vi "Insert CVT Data Core.vi"(4 "Data":variant, 5 "Nested Group":string, 6 "Nested?":bool, 7 "error in":errorcluster, 8 "tag":string, 9 "Group":string, 10 "CVT In":variant) -> (0 "error out":errorcluster, 3 "CVT Out":variant)   [LabVIEW 2014, in "Controller.lvlib" / "Controller.lvclass"]
uses:
  Controller.lvclass
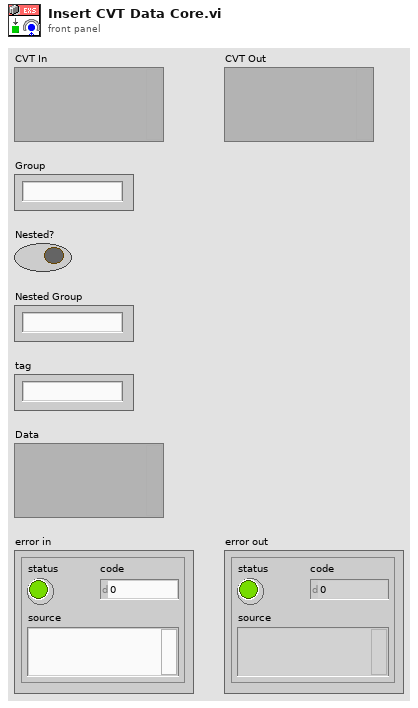
[diagram p1: front panel]
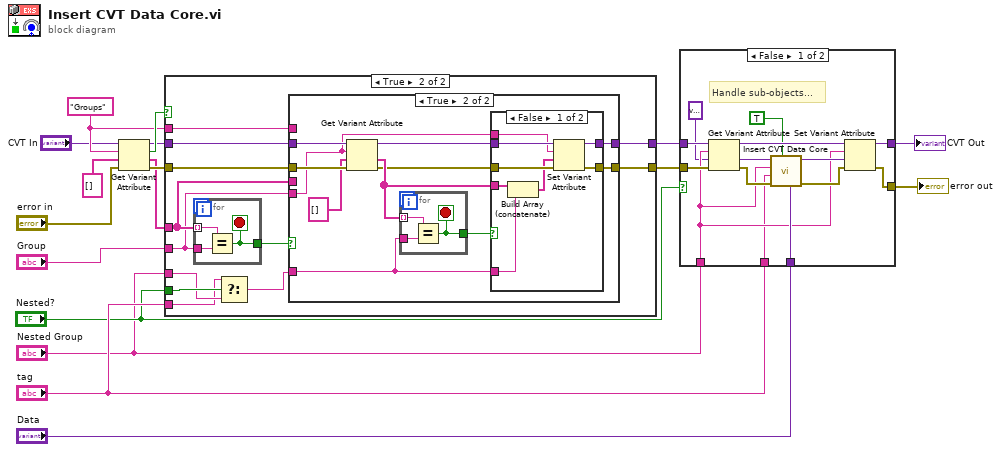
[diagram p0: block diagram]
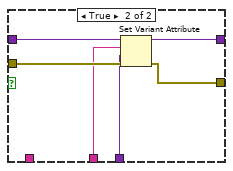
[diagram p2: hidden frame]
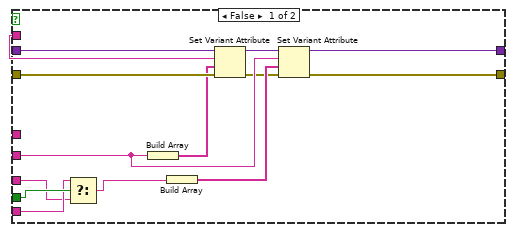
[diagram p3: hidden frame]
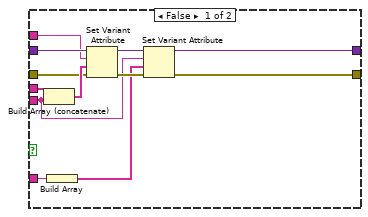
[diagram p4: hidden frame]
diagram:
  w7 = "Groups" ("name")
  n1 = Get Variant Attribute(Variant="CVT In", name=w7, default value (empty Variant)=string[] [], error in="error in") -> (duplicate Variant=w4:variant, found=w15:bool, value=w5:string[], error out=w8:errorcluster)
  n2 = case shown="True" w15 {
    tunnel: w4 -> [w31 w42]
    tunnel: w5 -> [_ w41]
    tunnel: "Group" -> [w25 w40]
    tunnel: w7 -> [w29 w39]
    tunnel: w8 -> [w30 w38]
    tunnel: [w26 w37] -> w9
    tunnel: [w23 w36] -> w10
    tunnel: "tag" -> [w20 w33]
    tunnel: "Nested?" -> [w21 w35]
    tunnel: "Nested Group" -> [w19 w34]
    frame False {
      n3 = Select(t=w20, s=w21, f=w19) -> (s? t:f=w18:string)
      n4 = Build Array(w25) -> (w28:string[])
      n5 = Build Array(w18) -> (w24:string[])
      n6 = Set Variant Attribute(Variant=w31, name=w29, value=w28, error in=w30) -> (Variant out=w27:variant, error out=w22:errorcluster)  [unwired: 1 out]
      n7 = Set Variant Attribute(Variant=w27, name=w25, value=w24, error in=w22) -> (Variant out=w26:variant, error out=w23:errorcluster)  [unwired: 1 out]
    }
    frame True {
      n8 = for {
        tunnel: w41 -> [w81] mode=indexing
        tunnel: w40 -> [w82]
        tunnel: [w80] -> w43
        stop <- w80 stop-if-true
        n9 = Equal?(x=w81, y=w82) -> (x = y?=w80:bool)
      }
      n10 = Select(t=w33, s=w35, f=w34) -> (s? t:f=w32:string)
      n11 = case shown="True" w43 {
        tunnel: w42 -> [w55 w66]
        tunnel: w41 -> [w54 _]
        tunnel: w40 -> [w48 w56]
        tunnel: w39 -> [w52 _]
        tunnel: [w45 w57] -> w37
        tunnel: [w44 w58] -> w36
        tunnel: w38 -> [w51 w65]
        tunnel: w32 -> [w47 w60]
        frame False {
          n12 = Build Array (concatenate)(w54, w48) -> (w53:string[])
          n13 = Build Array(w47) -> (w46:string[])
          n14 = Set Variant Attribute(Variant=w55, name=w52, value=w53, error in=w51) -> (Variant out=w50:variant, error out=w49:errorcluster)  [unwired: 1 out]
          n15 = Set Variant Attribute(Variant=w50, name=w48, value=w46, error in=w49) -> (Variant out=w45:variant, error out=w44:errorcluster)  [unwired: 1 out]
        }
        frame True {
          n16 = Get Variant Attribute(Variant=w66, name=w56, default value (empty Variant)=string[] [], error in=w65) -> (duplicate Variant=w62:variant, value=w61:string[], error out=w59:errorcluster)  [unwired: 1 out]
          n17 = for {
            tunnel: w61 -> [w78] mode=indexing
            tunnel: w60 -> [w79]
            tunnel: [w77] -> w63
            stop <- w77 stop-if-true
            n18 = Equal?(x=w78, y=w79) -> (x = y?=w77:bool)
          }
          n19 = case shown="False" w63 {
            tunnel: w62 -> [w74 w76]
            tunnel: w61 -> [w73 _]
            tunnel: w60 -> [w72 _]
            tunnel: w59 -> [w71 w75]
            tunnel: [w70 w75] -> w58
            tunnel: [w69 w76] -> w57
            tunnel: w56 -> [w67 _]
            frame False {
              n20 = Build Array (concatenate)(w73, w72) -> (w68:string[])
              n21 = Set Variant Attribute(Variant=w74, name=w67, value=w68, error in=w71) -> (Variant out=w69:variant, error out=w70:errorcluster)  [unwired: 1 out]
            }
            frame True {
            }
          }
        }
      }
    }
  }
  n22 = case shown="False" "Nested?" {
    tunnel: w9 -> [w96 w102]
    tunnel: w10 -> [w95 w101]
    tunnel: "Data" -> [w89 w100]
    tunnel: [w93 w99] -> w13
    tunnel: "tag" -> [w84 w98]
    tunnel: [w92 w97] -> w17
    tunnel: "Nested Group" -> [w85 _]
    frame False {
      # "Handle sub-objects..."
      n23 = Get Variant Attribute(Variant=w96, name=w85, default value (empty Variant)=variant ("default value (empty variant)"), error in=w95) -> (duplicate Variant=w94:variant, value=w91:variant, error out=w87:errorcluster)  [unwired: 1 out]
      n24 = call "Insert CVT Data Core.vi"("Data"=w89, "Nested?"=TRUE, "error in"=w87, "tag"=w84, "Group"=w85, "CVT In"=w91) -> ("error out"=w86:errorcluster, "CVT Out"=w90:variant)  [unwired: 3 in]
      n25 = Set Variant Attribute(Variant=w94, name=w85, value=w90, error in=w86) -> (Variant out=w93:variant, error out=w92:errorcluster)  [unwired: 1 out]
    }
    frame True {
      n26 = Set Variant Attribute(Variant=w102, name=w98, value=w100, error in=w101) -> (Variant out=w99:variant, error out=w97:errorcluster)  [unwired: 1 out]
    }
  }
  "error out" <- w17
  "CVT Out" <- w13
